vi "Set Waveform Display Intensity.vi"(8 "error in (no error)":errorcluster, 10 "Intensity (1-100)":i8=1 min=1 max=100 step=1, 11 "PicoScope 3000a in":refnum<class "PicoScope 3000a.lvclass">) -> (0 "error out":errorcluster, 3 "PicoScope 3000a out":refnum<class "PicoScope 3000a.lvclass">)   [LabVIEW 2018, in "PicoScope 3000a.lvlib" / "PicoScope 3000a.lvclass"]
doc: "This Override is used to change the display intensity level for the oscilloscope waveforms."
uses:
  PicoScope 3000a.lvclass
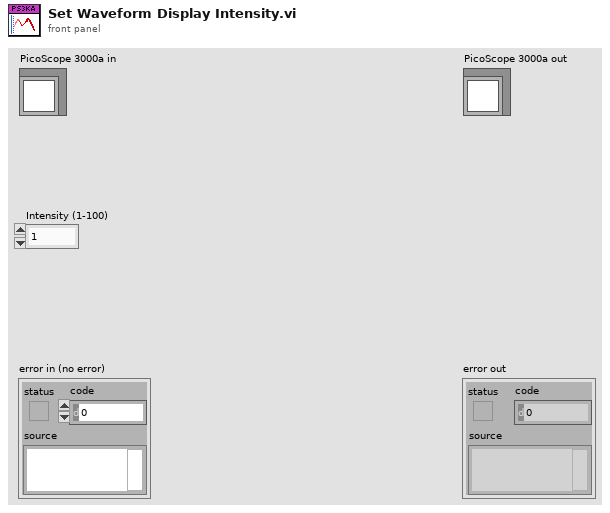
[diagram p1: front panel]
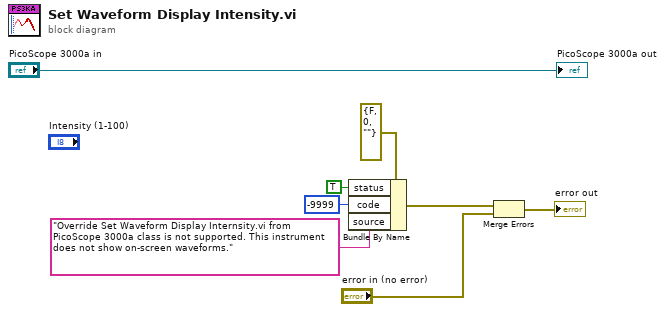
[diagram p0: block diagram]
diagram:
  n1 = Bundle By Name(cluster=errorcluster {"status"=FALSE, "code"=0, "source"=""} ("error constant"), "status"=TRUE, "code"=-9999, "source"="Override Set Waveform Display Internsity.vi from PicoScope 3000a class is not supported. This instrument does not show on-screen waveforms.") -> (w4:errorcluster)
  n2 = Merge Errors(w4, "error in (no error)") -> (→"error out":errorcluster)
  "PicoScope 3000a out" <- "PicoScope 3000a in"
